vi "Terminal-LoadSpectrum-InitQueue.vi"   [LabVIEW 2014]
types:
  T1 = enum16{"正常", "内部异常", "修改载荷谱", "外部异常", "外部停止", "其他"}
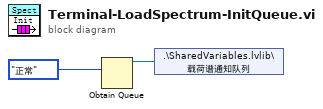
[diagram p0: block diagram]
diagram:
  n1 = Obtain Queue(element data type=T1."正常") -> (queue out=w1:refnum<queue>)  [unwired: 4 in, 2 out]
  n2 = shared-variable ".\\SharedVariables.lvlib\\载荷谱通知队列"(w1) -> ()  [unwired: 1 in, 1 out]
